vi "xijk_combined_single_file_reader.vi"(8 "error in (no error)":errorcluster, 9 "channel":string, 10 "element":string="#EX", 11 "file path input":path) -> (0 "error out":errorcluster, 3 "file path out":path)   [LabVIEW 2009, in "xijk_combined_file.lvlib"]
uses:
  xijk_combined_file.lvlib
  <vilib>/Utility/file.llb/Read From Spreadsheet File (string).vi
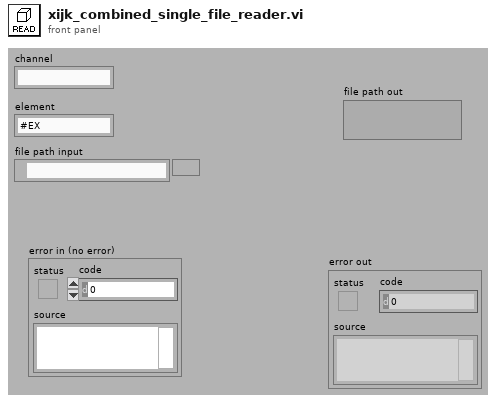
[diagram p1: front panel]
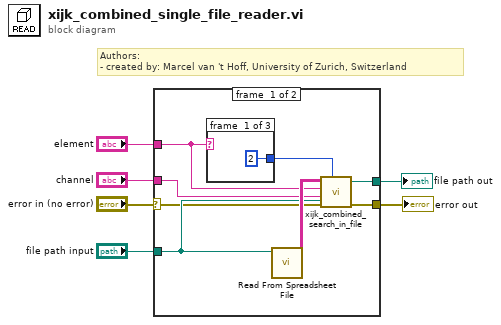
[diagram p0: block diagram]
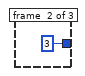
[diagram p2: hidden frame]
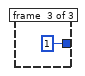
[diagram p3: hidden frame]
diagram:
  # "Authors: \n- created by: Marcel van 't Hoff, University of Zurich, Switzerland"
  n1 = case shown="No Error" "error in (no error)" {
    selector: "error in (no error)" -> [w8 w19]
    tunnel: [w13 w18] -> w6
    tunnel: "file path input" -> [w9 w18]
    tunnel: "element" -> [w12 _]
    tunnel: "channel" -> [w10 _]
    tunnel: [w7 w19] -> w1
    frame #0 {
      n2 = case shown="\"#BS\"" w12 {
        tunnel: [2 3 1] -> w11
        frame #0 {
        }
        frame #1 {
        }
        frame #2 {
        }
      }
      n3 = call-poly <vilib>:"Read From Spreadsheet File.vi"("file path (dialog if empty)"=w9) -> ("all rows"=w14:string[][])  [unwired: 6 in, 4 out]
      n4 = call "xijk_combined_search_in_file.vi"("file path in"=w9, "index (col)"=w11, "error in (no error)"=w8, "channel"=w10, "search input"=w12, "search 2D array"=w14) -> ("error out"=w7:errorcluster, "file path out"=w13:path)  [unwired: 4 in]
    }
    frame #1 {
    }
  }
  "file path out" <- w6
  "error out" <- w1
